vi "Test App Panels.vi"(8 "error in (no error)":errorcluster, 11 "GVIWebProcessorApp in":refnum<class "GVIWebProcessorApp.lvclass">) -> (0 "error out":errorcluster, 2 "PanelArray":refnum<class "ArrayManager.lvclass">, 3 "GVIWebProcessorApp out":refnum<class "GVIWebProcessorApp.lvclass">)   [LabVIEW 2020, in "PicoG-Processor.lvlib" / "GVIWebProcessorApp.lvclass"]
uses:
  GVIWebProcessorApp.lvclass
  <vilib>/IlluminatedG/IG OOPanel/OOPanel/ArrayManager/ArrayManager.lvclass
  WebProjectPanel/WebProjectPanel.lvclass
  C:/Program Files (x86)/National Instruments/LabVIEW 2020/vi.lib/IlluminatedG/IG OOPanel/OOPanel/ArrayPanel/ArrayPanel.lvclass
  GVIWebProcessorApp.lvclass/GVIWebProcessorApp.ctl
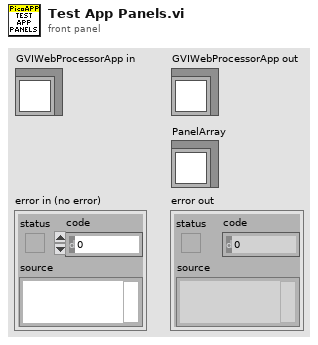
[diagram p1: front panel]
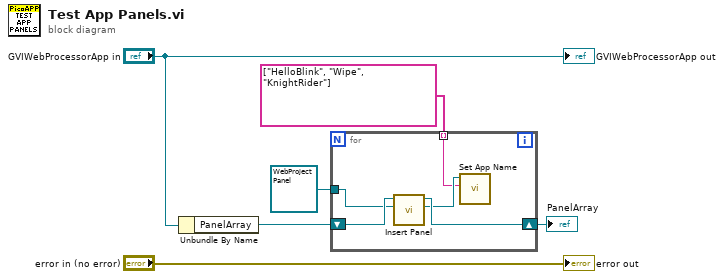
[diagram p0: block diagram]
diagram:
  n1 = Unbundle By Name("GVIWebProcessorApp in") -> ("PanelArray"=w2:refnum<class "ArrayManager.lvclass">)
  n2 = for {
    shift-right: [w11] -> w1
    shift-left: w2 -> [w10]
    tunnel: refnum<class "WebProjectPanel.lvclass"> refnum ("PicoG-Processor:WebProjectPanel.lvclass") -> [w9]
    tunnel: string[] ["HelloBlink", "Wipe", "KnightRider"] -> [w7] mode=indexing
    n3 = call <vilib>:"Insert Panel.vi"("Panel/Type"=w9, "PanelArray in"=w10) -> ("Panel"=w8:refnum<class "WebProjectPanel.lvclass">, "PanelArray out"=w11:refnum<class "ArrayManager.lvclass">)  [unwired: 7 in, 1 out]
    n4 = call "Set App Name.vi"("App Name"=w7, "WebProjectPanel in"=w8) -> ()  [unwired: 8 in, 2 out]
  }
  "PanelArray" <- w1
  "error out" <- "error in (no error)"
  "GVIWebProcessorApp out" <- "GVIWebProcessorApp in"
